vi "hydraharp_parse_TTR_records.vi"(7 "num_channels":i32=4, 8 "error in (no error)":errorcluster, 9 "Resolution":dbl=1.0, 10 "Mode":T1=2 items=["T2"=2, "T3"=3], 11 "fifo_buffer":u32[](array[numeric])) -> (0 "error out":errorcluster, 1 "channel_indices_in_buffer":i32[][](array[numeric]), 2 "photons_per_channel":i32[](array[numeric]), 3 "formatted_records":dbl[][](array[numeric]))   [LabVIEW 2015, in "hydraharp.lvclass"]
uses:
  hydraharp.lvclass
  hydraharp_panel/hpanel_acq_modes.ctl
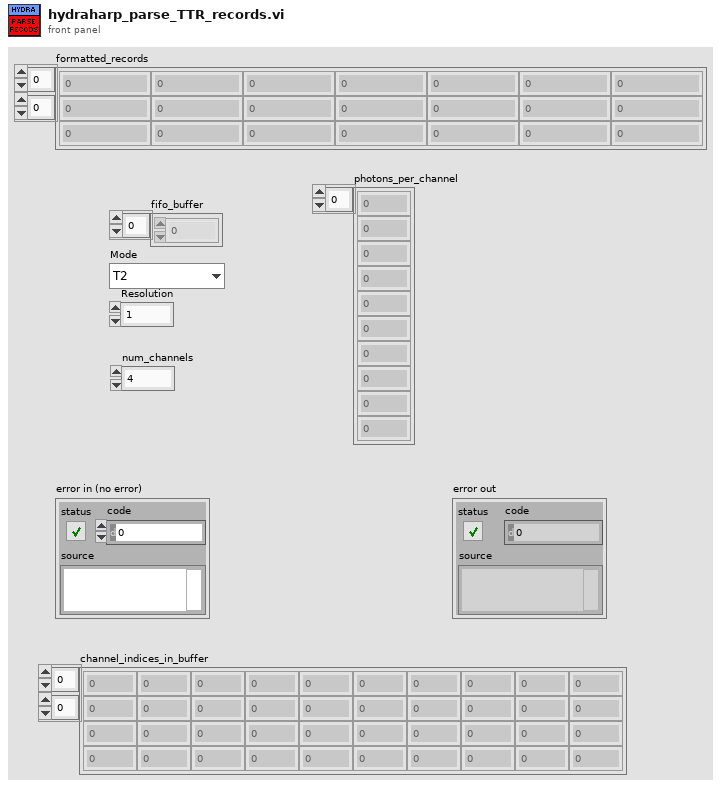
[diagram p1: front panel]
types:
  T1 = typedef "hpanel_acq_modes.ctl" = u16
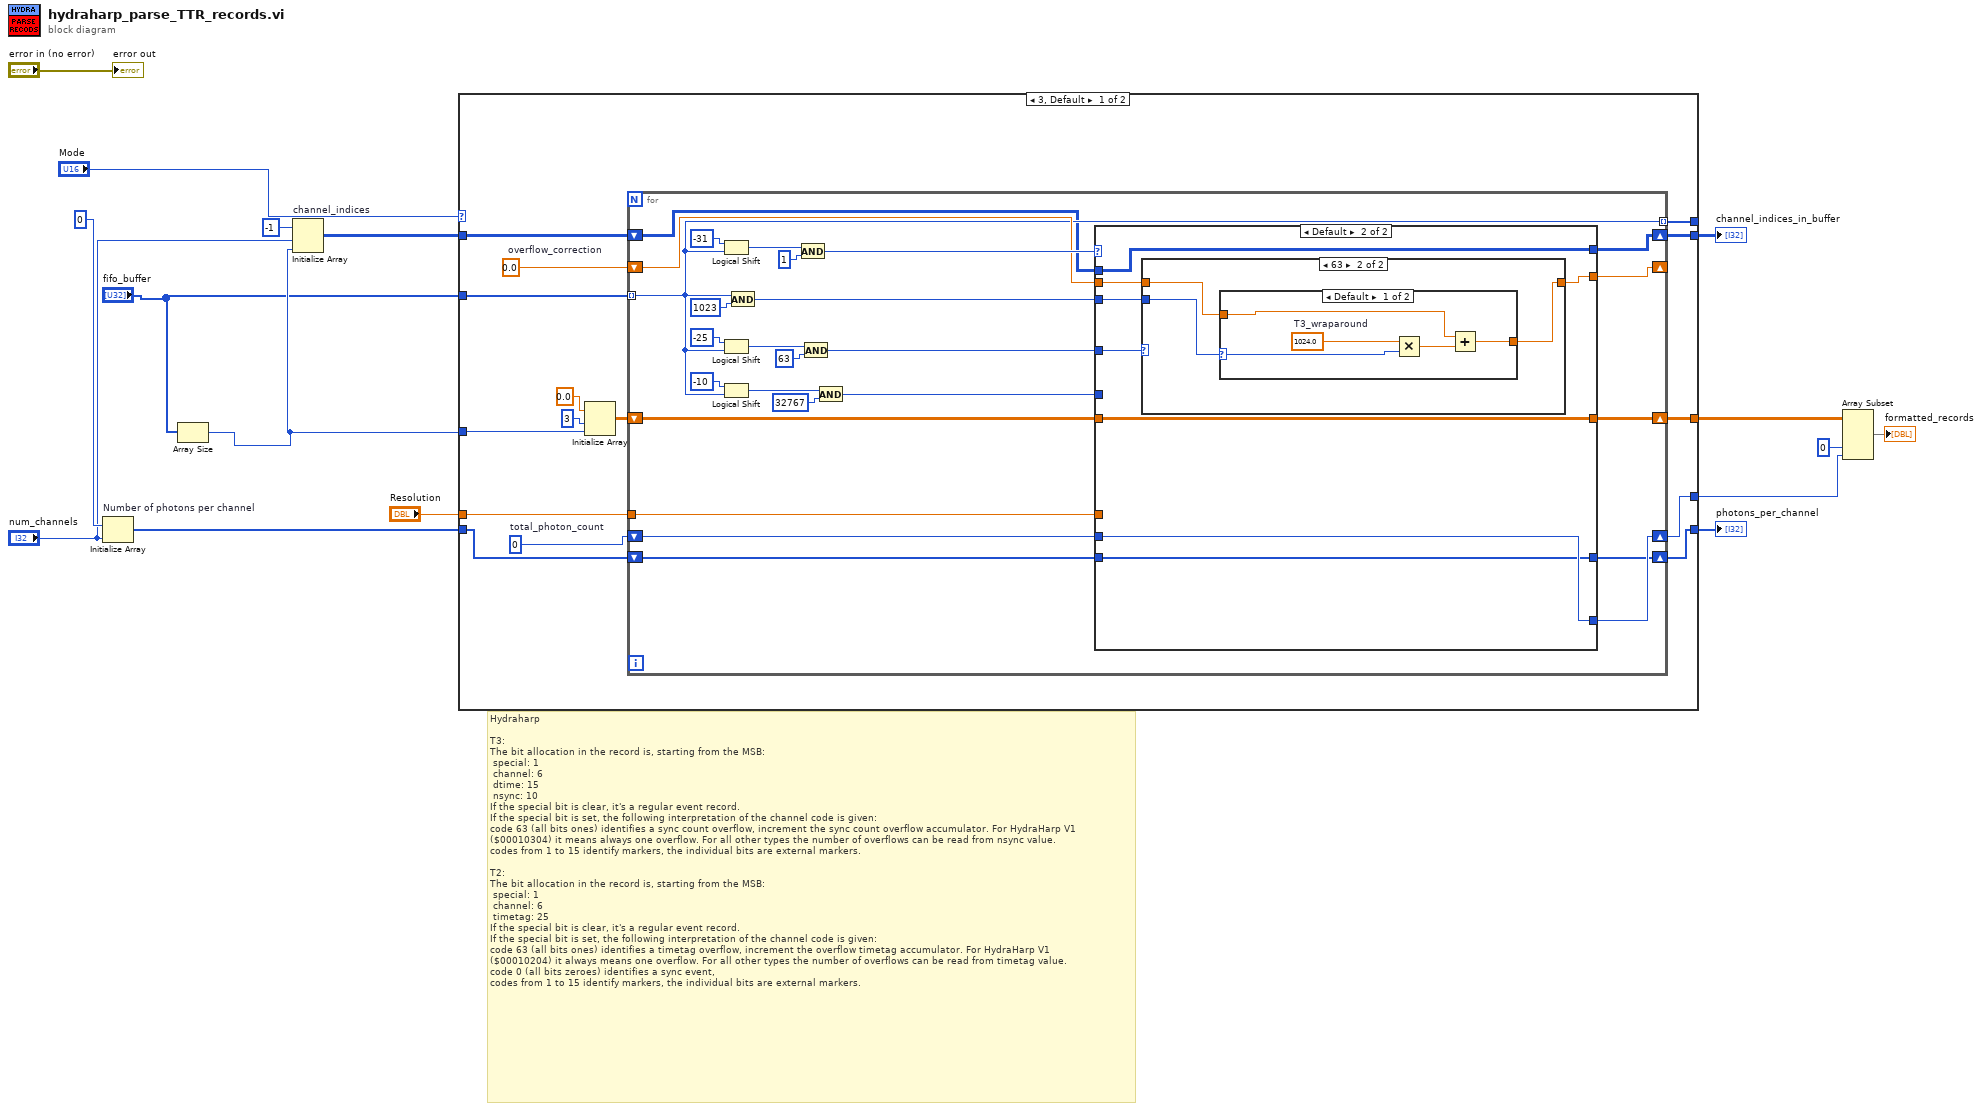
[diagram p0: block diagram]
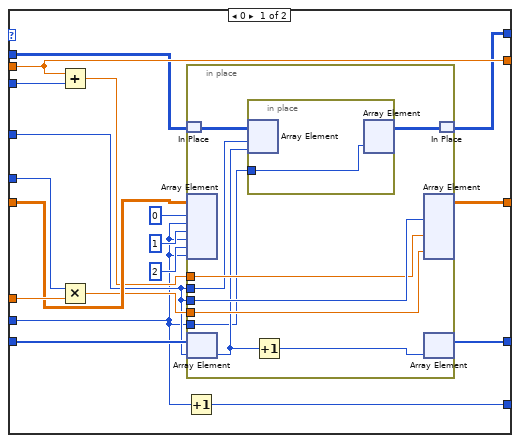
[diagram p2: hidden frame]
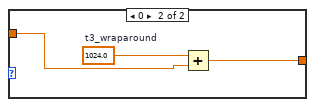
[diagram p4: hidden frame]
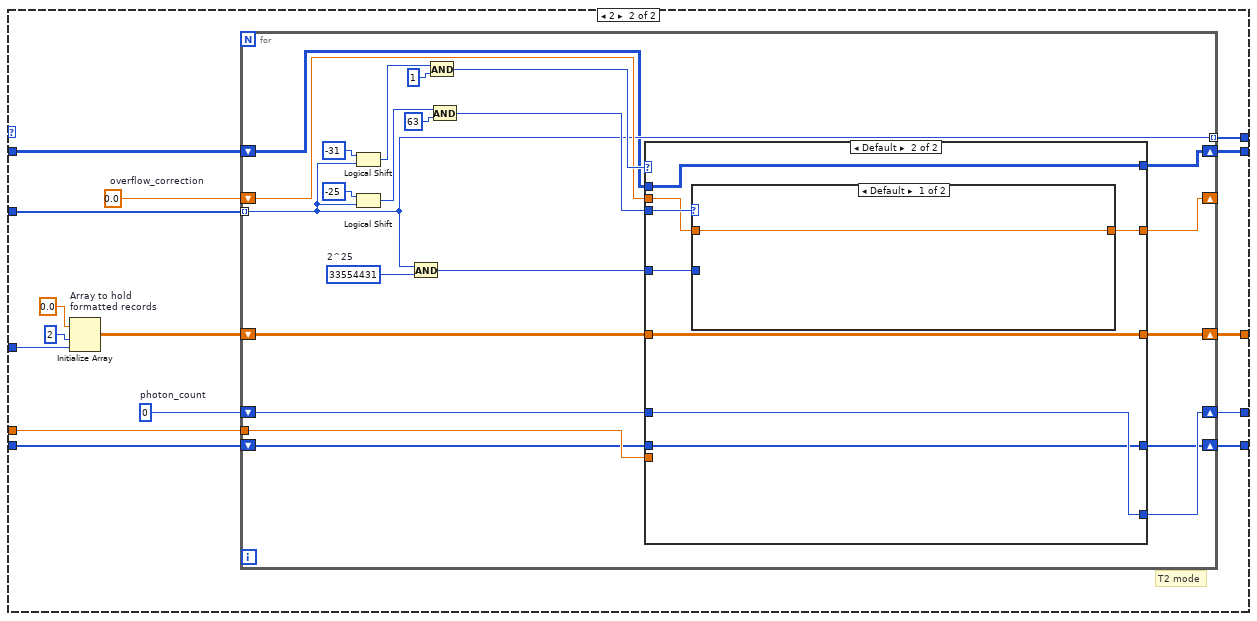
[diagram p5: hidden frame]
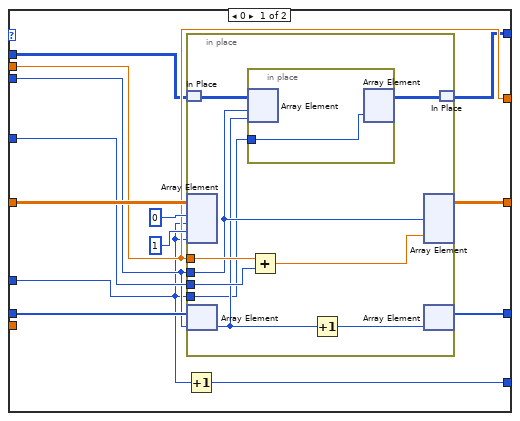
[diagram p6: hidden frame]
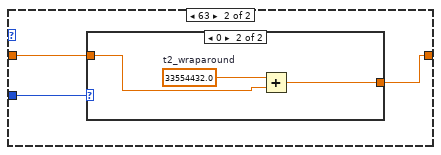
[diagram p7: hidden frame]
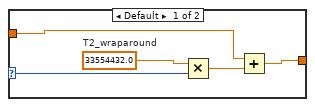
[diagram p8: hidden frame]
diagram:
  # "Hydraharp\n\nT3:\nThe bit allocation in the record is, starting from the MSB:\n special: 1\n channel: 6\n dtime: 15\n nsync: 10\nIf the special bit is clear, it's a regular event record.\nIf the special bit is set, the following interpretation of the channel code is given:\ncode 63 (all bits ones) identifies a sync count overflow, increment the sync count overflow accumulator. For HydraHarp V1\n($00010304) it means always one overflow. For all other types the number of overflows can be read from nsync value.\ncodes from 1 to 15 identify markers, the individual bits are external markers.\n\nT2: \nThe bit allocation in the record is, starting from the MSB:\n special: 1\n channel: 6\n timetag: 25\nIf the special bit is clear, it's a regular event record.\nIf the special bit is set, the following interpretation of the channel code is given:\ncode 63 (all bits ones) identifies a timetag overflow, increment the overflow timetag accumulator. For HydraHarp V1\n($00010204) it always means one overflow. For all other types the number of overflows can be read from timetag value.\ncode 0 (all bits zeroes) identifies a sync event,\ncodes from 1 to 15 identify markers, the individual bits are external markers."
  n1 = Initialize Array "Number of photons per channel"(0 ("element"), "num_channels") -> (w10:i32[])
  n2 = Array Size(array="fifo_buffer") -> (size(s)=w2:i32)
  n3 = Initialize Array "channel_indices"(-1 ("element"), "num_channels", w2) -> (w5:i32[][])
  n4 = case shown="3, Default" "Mode" {
    tunnel: "fifo_buffer" -> [w30 w119]
    tunnel: [w25 w114] -> _
    tunnel: "Resolution" -> [w24 w113]
    tunnel: [w23 w112] -> w15
    tunnel: [w22 w111] -> w13
    tunnel: w10 -> [w21 w110]
    tunnel: [w20 w109] -> w9
    tunnel: w2 -> [w19 w108]
    tunnel: w5 -> [w18 w107]
    tunnel: [w17 w106] -> w4
    frame 3, Default {
      w26 = 0  # total_photon_count
      w27 = 0.0  # overflow_correction
      n5 = Initialize Array(0.0 ("element"), 3 ("dimension size"), w19) -> (w28:dbl[][])
      n6 = for {
        tunnel: w30 -> [w36] mode=indexing
        shift-right: [w39] -> w23
        shift-left: w28 -> [w46]
        shift-right: [w37] -> _
        shift-left: w27 -> [w45]
        tunnel: w24 -> [w42]
        shift-right: [w38] -> w22
        shift-left: w26 -> [w40]
        tunnel: [w36] -> w25 mode=indexing
        shift-right: [w34] -> w20
        shift-left: w21 -> [w35]
        shift-right: [w32] -> w17
        shift-left: w18 -> [w33]
        n7 = Logical Shift(y=i16 -31, x=w36) -> (x << y=w49:u32)
        n8 = Logical Shift(y=i16 -25, x=w36) -> (x << y=w52:u32)
        n9 = Logical Shift(y=i16 -10, x=w36) -> (x << y=w55:u32)
        n10 = And(x=w36, y=u32 1023) -> (x .and. y?=w44:u32)
        n11 = And(x=w49, y=u32 1) -> (x .and. y?=w47:u32)
        n12 = And(x=w52, y=u32 63) -> (x .and. y?=w41:u32)
        n13 = And(x=w55, y=u32 32767) -> (x .and. y?=w43:u32)
        n14 = case shown="Default" w47 {
          tunnel: w46 -> [w72 w88]
          tunnel: w45 -> [w64 w91]
          tunnel: w44 -> [w75 w92]
          tunnel: w43 -> [w73 _]
          tunnel: w42 -> [w74 _]
          tunnel: w41 -> [w59 w93]
          tunnel: w40 -> [w58 w89]
          tunnel: [w66 w88] -> w39
          tunnel: [w65 w89] -> w38
          tunnel: [w64 w90] -> w37
          tunnel: w35 -> [w63 w87]
          tunnel: [w62 w87] -> w34
          tunnel: w33 -> [w61 w86]
          tunnel: [w60 w86] -> w32
          frame 0 {
            n15 = Add(x=w64, y=w75) -> (x+y=w68:dbl)
            n16 = Multiply(x=w73, y=w74) -> (x*y=w67:dbl)
            n17 = Increment(x=w58) -> (x+1=w65:i32)
            n18 = in-place {
              in-place-border: w59 -> [w84]
              in-place-border: w68 -> [w83]
              in-place-border: w67 -> [w82]
              in-place-border: w59 -> [w79]
              in-place-border: w58 -> [w77]
              n19 = in-place-match #1(w61) -> (w80:i32[][])
              n20 = in-place-array #2(w72, 0, w58, 1, w58, 2, w58) -> ()  [unwired: 3 out]
              n21 = in-place-array #3(w63, w59) -> (w78:i32)
              n22 = in-place {
                in-place-border: w77 -> [w85]
                n23 = in-place-array #4(w80, w79, w78) -> ()  [unwired: 1 out]
                n24 = in-place-array #4(w85) -> (w76:i32[][])  [unwired: 2 out]
              }
              n25 = Increment(x=w78) -> (x+1=w81:i32)
              n26 = in-place-array #2(w84, w83, w82) -> (w66:dbl[][])  [unwired: 6 out]
              n27 = in-place-array #3(w81) -> (w62:i32[])  [unwired: 1 out]
              n28 = in-place-match #1(w76) -> (w60:i32[][])
            }
          }
          frame Default {
            n29 = case shown="63" w93 {
              tunnel: w92 -> [_ w97]
              tunnel: w91 -> [w94 w96]
              tunnel: [w94 w95] -> w90
              frame Default {
              }
              frame 63 {
                n30 = case shown="Default" w97 {
                  selector: w97 -> [w100 _]
                  tunnel: w96 -> [w102 w105]
                  tunnel: [w98 w103] -> w95
                  frame Default {
                    w101 = 1024.0  # T3_wraparound
                    n31 = Multiply(x=w101, y=w100) -> (x*y=w99:dbl)
                    n32 = Add(x=w102, y=w99) -> (x+y=w98:dbl)
                  }
                  frame 0 {
                    w104 = 1024.0  # t3_wraparound
                    n33 = Add(x=w104, y=w105) -> (x+y=w103:dbl)
                  }
                }
              }
            }
          }
        }
      }
    }
    frame 2 {
      w115 = 0  # photon_count
      w116 = 0.0  # overflow_correction
      # "T2 mode"
      n34 = Initialize Array "Array to hold\nformatted records"(0.0 ("element"), 2 ("dimension size"), w108) -> (w117:dbl[][])
      n35 = for {
        tunnel: w119 -> [w125] mode=indexing
        shift-right: [w128] -> w112
        shift-left: w117 -> [w134]
        shift-right: [w126] -> _
        shift-left: w116 -> [w133]
        tunnel: w113 -> [w131]
        shift-right: [w127] -> w111
        shift-left: w115 -> [w129]
        tunnel: [w125] -> w114 mode=indexing
        shift-right: [w123] -> w109
        shift-left: w110 -> [w124]
        shift-right: [w121] -> w106
        shift-left: w107 -> [w122]
        w142 = u32 33554431  # 2^25
        n36 = Logical Shift(y=i16 -31, x=w125) -> (x << y=w137:u32)
        n37 = Logical Shift(y=i16 -25, x=w125) -> (x << y=w140:u32)
        n38 = And(x=w125, y=w142) -> (x .and. y?=w132:u32)
        n39 = And(x=w137, y=u32 1) -> (x .and. y?=w135:u32)
        n40 = And(x=w140, y=u32 63) -> (x .and. y?=w130:u32)
        n41 = case shown="Default" w135 {
          tunnel: w134 -> [w155 w168]
          tunnel: w133 -> [w151 w171]
          tunnel: w132 -> [w150 w172]
          tunnel: w131 -> [_ _]
          tunnel: w130 -> [w147 w173]
          tunnel: w129 -> [w143 w169]
          tunnel: [w152 w168] -> w128
          tunnel: [w145 w169] -> w127
          tunnel: [w151 w170] -> w126
          tunnel: w124 -> [w149 w167]
          tunnel: [w148 w167] -> w123
          tunnel: w122 -> [w146 w166]
          tunnel: [w144 w166] -> w121
          frame 0 {
            n42 = Increment(x=w143) -> (x+1=w145:i32)
            n43 = in-place {
              in-place-border: w147 -> [w159]
              in-place-border: w151 -> [w164]
              in-place-border: w150 -> [w163]
              in-place-border: w143 -> [w157]
              n44 = in-place-match #5(w146) -> (w160:i32[][])
              n45 = in-place-array #6(w155, 0, w143, 1, w143) -> ()  [unwired: 2 out]
              n46 = in-place-array #7(w149, w147) -> (w158:i32)
              n47 = in-place {
                in-place-border: w157 -> [w165]
                n48 = in-place-array #8(w160, w159, w158) -> ()  [unwired: 1 out]
                n49 = in-place-array #8(w165) -> (w156:i32[][])  [unwired: 2 out]
              }
              n50 = Add(x=w164, y=w163) -> (x+y=w162:dbl)
              n51 = Increment(x=w158) -> (x+1=w161:i32)
              n52 = in-place-array #6(w159, w162) -> (w152:dbl[][])  [unwired: 4 out]
              n53 = in-place-array #7(w161) -> (w148:i32[])  [unwired: 1 out]
              n54 = in-place-match #5(w156) -> (w144:i32[][])
            }
          }
          frame Default {
            n55 = case shown="Default" w173 {
              tunnel: w172 -> [_ w177]
              tunnel: w171 -> [w174 w176]
              tunnel: [w174 w175] -> w170
              frame Default {
              }
              frame 63 {
                n56 = case shown="0" w177 {
                  selector: w177 -> [w180 _]
                  tunnel: w176 -> [w182 w185]
                  tunnel: [w178 w183] -> w175
                  frame Default {
                    w181 = 33554432.0  # T2_wraparound
                    n57 = Multiply(x=w181, y=w180) -> (x*y=w179:dbl)
                    n58 = Add(x=w182, y=w179) -> (x+y=w178:dbl)
                  }
                  frame 0 {
                    w184 = 33554432.0  # t2_wraparound
                    n59 = Add(x=w184, y=w185) -> (x+y=w183:dbl)
                  }
                }
              }
            }
          }
        }
      }
    }
  }
  "photons_per_channel" <- w9
  "channel_indices_in_buffer" <- w4
  n60 = Array Subset(array=w15, index (col)=0 ("index"), length (col)=w13) -> (→"formatted_records":dbl[][])  [unwired: 2 in]
  "error out" <- "error in (no error)"
